vi "Set Payload DVR.vi"(7 "Msg":refnum<class "Msg.lvclass">, 11 "Payload DVR":refnum<data-value>) -> (5 "Msg":refnum<class "Msg.lvclass">)   [LabVIEW 2020, in "_Template.lvlib" / "{{Msg}}.lvlib" / "Msg.lvclass"]
uses:
  Msg.lvclass
  Msg.lvclass/Msg.ctl
  Payload.ctl
  {{Msg}}.lvlib
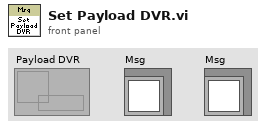
[diagram p1: front panel]
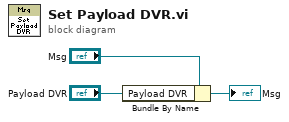
[diagram p0: block diagram]
diagram:
  n1 = Bundle By Name(cluster="Msg", "Payload DVR"="Payload DVR") -> (→"Msg":refnum<class "Msg.lvclass">)
